vi "SET_BURGLAR.vi"(10 "argv":string[](array[string]), 11 "args":u8) -> ()   [LabVIEW 2015]
uses:
  Team Code/Robot Global Data.vi
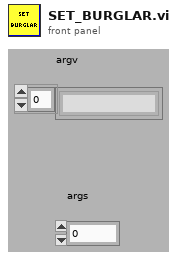
[diagram p1: front panel]
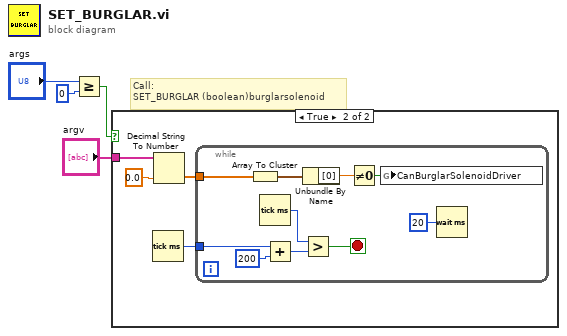
[diagram p0: block diagram]
diagram:
  # "Call:\nSET_BURGLAR (boolean)burglarsolenoid"
  n1 = Greater Or Equal?(x="args", y=u8 0) -> (x >= y?=w4:bool)
  n2 = case shown="True" w4 {
    tunnel: "argv" -> [_ w8]
    frame False {
    }
    frame True {
      n3 = Tick Count (ms)() -> (millisecond timer value=w5:u32)
      n4 = Decimal String To Number(string=w8, default (0L)=0.0 ("default (0 I32)")) -> (number=w6:dbl[])  [unwired: 2 out]
      n5 = while {
        tunnel: w6 -> [w18]
        tunnel: w5 -> [w14]
        stop <- w10 stop-if-true
        n6 = Array To Cluster(array=w18) -> (cluster=w17:cluster{"[0]":dbl, "[1]":dbl})
        n7 = Tick Count (ms)() -> (millisecond timer value=w12:u32)
        n8 = Add(x=w14, y=u32 200) -> (x+y=w11:u32)
        n9 = Unbundle By Name(w17) -> ("[0]"=w16:dbl)
        n10 = Greater?(x=w12, y=w11) -> (0:w10:bool)
        n11 = Not Equal To 0?(x=w16) -> (x != 0?=w15:bool)
        n12 = global write "Robot Global Data.vi" "CanBurglarSolenoidDriver"(w15) -> ()
        n13 = Wait (ms)(milliseconds to wait=u32 20) -> ()  [unwired: 1 out]
      }
    }
  }
